vi "TestNewmarkOpenClose.vi"() -> ()   [LabVIEW 2020]
uses:
  <vilib>/Galil/resources/gclib32/gclib32.lvlib
panel:
  out "error out 2":errorcluster
  out "error out":errorcluster
  in  "error in (no error)":errorcluster
  in  "address":string="192.168.17.226"
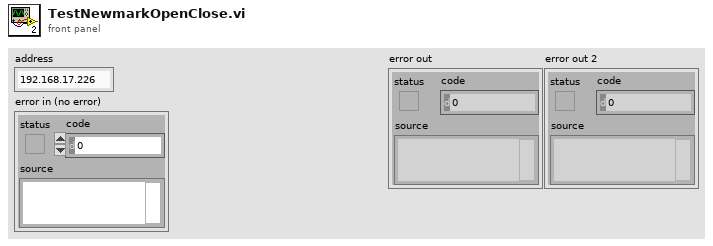
[diagram p1: front panel]
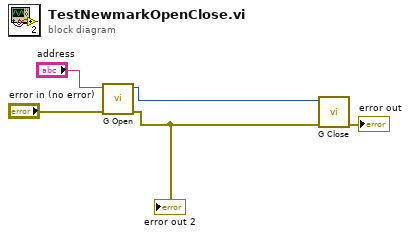
[diagram p0: block diagram]
diagram:
  n1 = call <vilib>:"G Open.vi"("error in (no error)"="error in (no error)", "address"="address") -> ("error out"=w3:errorcluster, "g out"=w2:u32)  [unwired: 7 in]
  "error out 2" <- w3
  n2 = call <vilib>:"G Close.vi"("error in (no error)"=w3, "g"=w2) -> ("error out"=→"error out":errorcluster)  [unwired: 9 in]
